vi "Test Copy Array To Image ARGBPixel.vi"(8 "error in (no error)":errorcluster, 11 "Test Case In":refnum<class "Image.lvclass">) -> (0 "error out":errorcluster, 3 "Test Case Out":refnum<class "Image.lvclass">)   [LabVIEW 2020, in "g_ar_toolkit.test.lvlib" / "Image.lvclass"]
uses:
  Image.lvclass
  C:/Program Files (x86)/National Instruments/LabVIEW 2020/vi.lib/Astemes/LUnit/Test Case.lvclass
  g_ar_toolkit.common/Image Size (Integer).ctl
  <vilib>/Astemes/LUnit/Test Case.lvclass/Test Case.ctl
  g_ar_toolkit.image/CreateEmptyImageARGB.vi
  4993e8ee-a06a-463a-9684-69129f64d5ce.vi
  g_ar_toolkit.image/Copy Array to Image.vi
  g_ar_toolkit.image/CopyArrayToImageARGB.vi
  g_ar_toolkit.image/CreateEmptyImageARGB.vi/3321fa97-f432-4e1e-8db9-a0df79aed21b.vi
  <vilib>/Astemes/LUnit/Append Pass Result.vi
  <vilib>/Astemes/LUnit/Append Fail Result.vi
  <vilib>/Astemes/LUnit/Describe Comparison.vi
  <vilib>/Astemes/LUnit/Compare Variants.vi
  g_ar_toolkit.image/CopyArrayToImageARGB.vi/26c70cee-9332-41f4-9755-08948a885cbe.vi
  <vilib>/Astemes/LUnit/Run In UI.vi
  <vilib>/Utility/error.llb/Clear Errors.vi
  g_ar_toolkit.image/ARGBColourToU32.vi
  g_ar_toolkit.common/Module Path.vi
  <vilib>/Utility/error.llb/Error Cluster From Error Code.vi
  <vilib>/picture/pixmap.llb/Flatten Pixmap.vi
  <vilib>/Astemes/LUnit/Describe Variant.vi
  Image.lvclass/Image.ctl
  g_ar_toolkit.image/g_ar_toolkit.image.lvlib
  g_ar_toolkit.common/g_ar_toolkit.common.lvlib
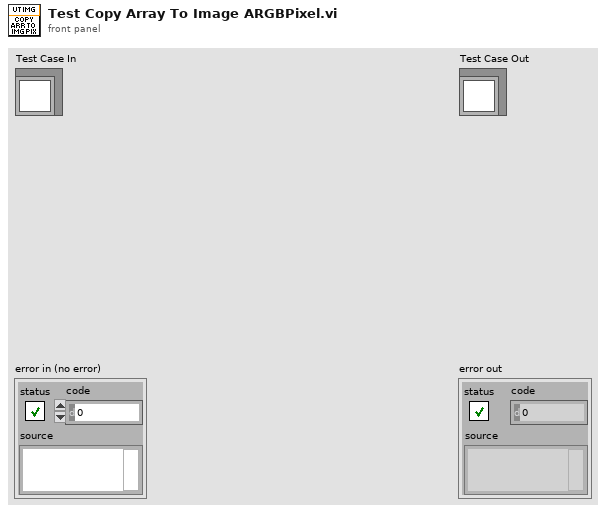
[diagram p1: front panel]
types:
  T1 = typedef "g_ar_toolkit.common.lvlib/Image Size (Integer).ctl" = cluster{"Width":u16, "Height":u16}
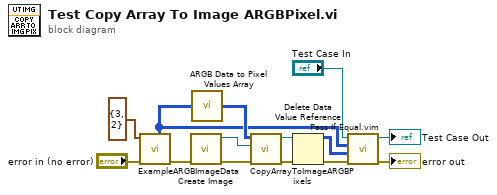
[diagram p0: block diagram]
diagram:
  n1 = call "ExampleARGBImageData.vi"("error in (no error)"="error in (no error)", "Image Size"=T1 {"Width"=3, "Height"=2}) -> ("error out"=w3:errorcluster, "ARGB Array Data"=w2:u32[][])  [unwired: 6 in, 2 out]
  n2 = call-poly "Create Image.vi"("error in (no error)"=w3) -> ("error out"=w9:errorcluster, "New ARGB Image"=w8:refnum<data-value>)  [unwired: 9 in]
  n3 = call "ARGB Data to Pixel Values Array.vi"("ARGB Data"=w2) -> ("Pixel Values"=w7:u8[][][])
  n4 = call "CopyArrayToImageARGBPixels.vi"("error in (no error)"=w9, "ARGB Image Destination"=w8, "Source"=w7) -> ("error out"=w6:errorcluster, "ARGB Image Destination (Duplicate)"=w5:refnum<data-value>)  [unwired: 7 in]
  n5 = Delete Data Value Reference(data value reference=w5, error in=w6) -> (data value=w11:u32[][], error out=w10:errorcluster)
  n6 = call "Pass If Equal.vim"("error in (no error)"=w10, "Actual"=w11, "Expected"=w2, "LUnit Test Case In"="Test Case In") -> ("error out"=→"error out":errorcluster, "LUnit Test Case Out"=→"Test Case Out":refnum<class "Image.lvclass">)  [unwired: 6 in]
